vi "Subscribe (Scalar).vi"(6 "timeout (1000ms)":i32=1000, 8 "error in (no error)":errorcluster, 9 "QoS":T1, 10 "Topic Filter":string, 11 "Client in":refnum<class "Client.lvclass">) -> (0 "error out":errorcluster, 1 "Ack":bool, 3 "Client out":refnum<class "Client.lvclass">)   [LabVIEW 2013, in "MQTT Client.lvlib" / "Client.lvclass"]
uses:
  Client.lvclass
  <vilib>/LabVIEW Open Source Project/MQTT Control Packets/Control Packets/ControlPacket/QualityOfService -- enum.ctl
  <vilib>/LabVIEW Open Source Project/MQTT Connection/MQTT_Base/Base Class/MQTT_Base.lvclass
  <vilib>/LabVIEW Open Source Project/MQTT Control Packets/Control Packets/ControlPacket/ControlPacket.lvclass
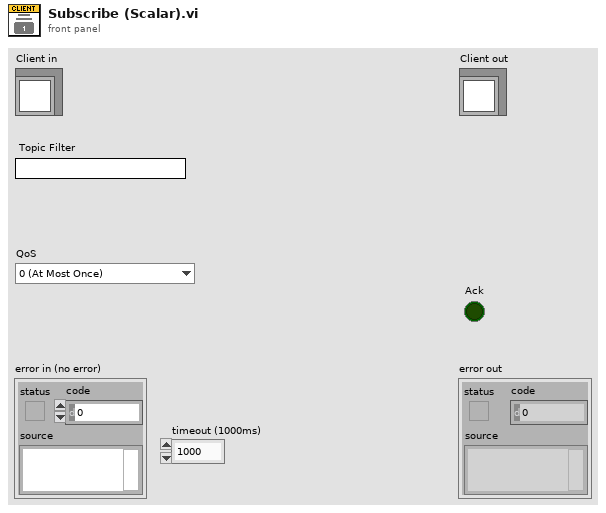
[diagram p1: front panel]
types:
  T1 = typedef "MQTT_Control_Packets.lvlib/ControlPacket.lvclass/QualityOfService -- enum.ctl" = enum16{"0 (At Most Once)", "1 (At Least Once)", "2 (Exactly Once)"}
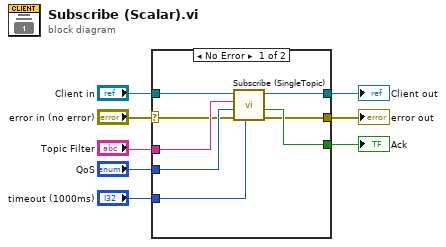
[diagram p0: block diagram]
diagram:
  n1 = case shown="No Error" "error in (no error)" {
    selector: "error in (no error)" -> [w10 w18]
    tunnel: [w9 w18] -> w7
    tunnel: [w15 w17] -> w5
    tunnel: "Client in" -> [w16 w17]
    tunnel: [w14 _] -> w4
    tunnel: "Topic Filter" -> [w13 _]
    tunnel: "QoS" -> [w12 _]
    tunnel: "timeout (1000ms)" -> [w11 _]
    frame No Error {
      n2 = call <vilib>:"Subscribe (SingleTopic).vi"("timeout (100ms)"=w11, "error in (no error)"=w10, "QoS"=w12, "Topic Filter"=w13, "MQTT_Base in"=w16) -> ("error out"=w9:errorcluster, "Ack"=w14:bool, "MQTT_Base out"=w15:refnum<class "Client.lvclass">)  [unwired: 4 in]
    }
    frame Error {
    }
  }
  "error out" <- w7
  "Client out" <- w5
  "Ack" <- w4
